vi "FGV_Connected-Axes.vi"(3 "error in":errorcluster, 4 "Conn. \nAxis in":string[](array[string]), 5 "Action":T1) -> (0 "error out":errorcluster, 1 "Conn. \nAxis out":string[](array[string]))   [LabVIEW 2026]
uses:
  TypeDef_FGV.ctl
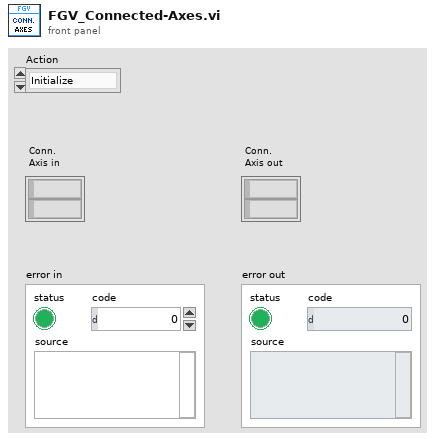
[diagram p1: front panel]
types:
  T1 = typedef "TypeDef_FGV.ctl" = enum16{"Initialize", "Write", "Read"}
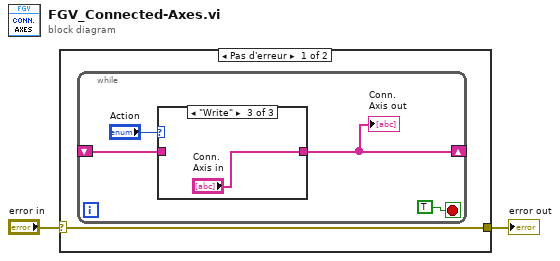
[diagram p0: block diagram]
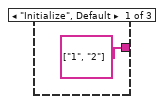
[diagram p2: hidden frame]
diagram:
  n1 = case shown="Pas d'erreur" "error in" {
    selector: "error in" -> [w3 w11]
    tunnel: [w3 w11] -> w2
    frame No Error {
      n2 = while {
        shift-right: [w4] -> _
        shift-left: _ -> [w5]
        stop <- TRUE stop-if-true
        n3 = case shown="\"Write\"" "Action" {
          tunnel: w5 -> [_ w9 _]
          tunnel: [string[] ["1", "2"] ("Conn. \nAxis") w9 "Conn. \nAxis in"] -> w4
          frame "Initialize", Default {
          }
          frame "Read" {
          }
          frame "Write" {
          }
        }
        "Conn. \nAxis out" <- w4
      }
    }
    frame Error {
    }
  }
  "error out" <- w2
